vi "Fix Sequence.vi"(0 "sequences":string[](array[string]), 1 "shots":string[](array[string]), 2 "old sequence list":string[][](array[string]), 3 "image_data":u16[][][](array[numeric]), 4 "keep?":bool) -> (5 "sequencer":T1(array[cluster]), 6 "held data":u16[][][](array[numeric]))   [LabVIEW 2010]
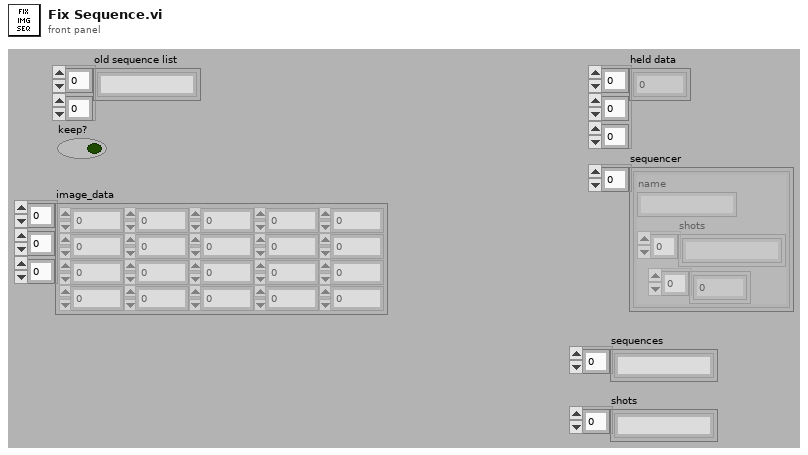
[diagram p1: front panel]
types:
  T1 = cluster{"name":string, "shots":string[], i32[]}[]
  T2 = cluster{"name":string, "shots":string[], "id":i32[]}[]
  T3 = cluster{"name":string, "kept frames":string[], i32[]}
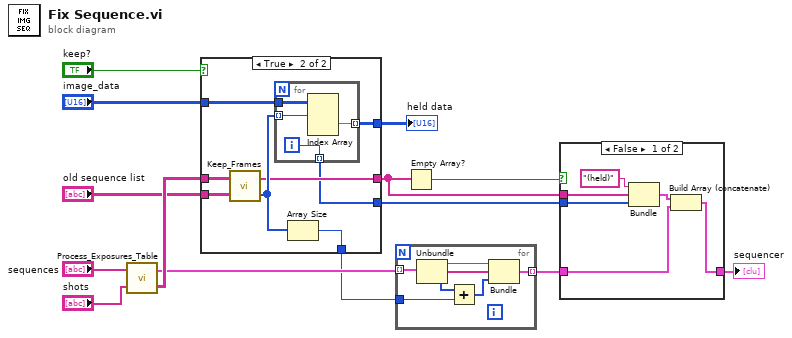
[diagram p0: block diagram]
diagram:
  n1 = call "Process_Exposures_Table.vi"("shot names"="shots", "sequence names"="sequences") -> ("list"=w14:string[][], "sequences"=w11:T2)
  n2 = case shown="True" "keep?" {
    tunnel: w14 -> [_ w18]
    tunnel: "old sequence list" -> [_ w22]
    tunnel: [_ w16] -> w4
    tunnel: [_ w21] -> w2
    tunnel: [_ w20] -> w10
    tunnel: "image_data" -> [_ w19]
    tunnel: [_ w15] -> w5
    frame False {
    }
    frame True {
      n3 = call "Keep_Frames.vi"("old list"=w22, "list"=w18) -> ("kept indices"=w17:i32[], "kept frames"=w16:string[])
      n4 = for {
        tunnel: w17 -> [w25] mode=indexing
        tunnel: w19 -> [w26]
        tunnel: [w24] -> w21 mode=indexing
        tunnel: [w23] -> w15 mode=indexing
        i -> [w23]
        n5 = Index Array(array=w26, index (dim 0)=w25) -> (element=w24:u16[][])  [unwired: 2 in]
      }
      n6 = Array Size(array=w17) -> (size(s)=w20:i32)
    }
  }
  "held data" <- w2
  n7 = for {
    tunnel: w11 -> [w33] mode=indexing
    tunnel: w10 -> [w28]
    tunnel: [w27] -> w6 mode=indexing
    n8 = Unbundle(w33) -> ("name"=w32:string, "shots"=w31:string[], "id"=w30:i32[])
    n9 = Add(x=w30, y=w28) -> (x+y=w29:i32[])
    n10 = Bundle("name"=w32, "shots"=w31, w29) -> (w27:cluster{"name":string, "shots":string[], i32[]})  [unwired: 1 in]
  }
  n11 = Empty Array?(array=w4) -> (empty?=w3:bool)
  n12 = case shown="False" w3 {
    tunnel: w5 -> [w39 _]
    tunnel: w4 -> [w38 _]
    tunnel: w6 -> [w35 w40]
    tunnel: [w34 w40] -> w1
    frame False {
      n13 = Bundle("name"="(held)", "kept frames"=w38, w39) -> (w36:T3)  [unwired: 1 in]
      n14 = Build Array (concatenate)(w36, w35) -> (w34:T1)
    }
    frame True {
    }
  }
  "sequencer" <- w1
